vi "Add Item Buffered.vi"(8 "错误输入":errorcluster, 9 "Length":i32=20, 10 "Item":string[](array[string]), 11 "Mlistbox Ref":refnum<vi>) -> (0 "错误输出":errorcluster, 3 "Mlistbox Ref Dup":refnum<vi>)   [LabVIEW 2012, in "Mlistbox Tools.lvlib"]
uses:
  Mlistbox Tools.lvlib
  ListBox/Custom Type/Read and Write Mode.ctl
  Property/Set and Get ItemNames.vi
  ListBox/Listbox Tool.lvlib
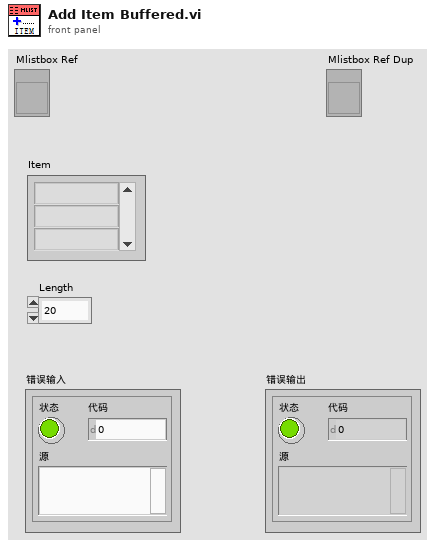
[diagram p1: front panel]
types:
  T1 = typedef "Listbox Tool.lvlib/Read and Write Mode.ctl" = enum16{"Read", "Write"}
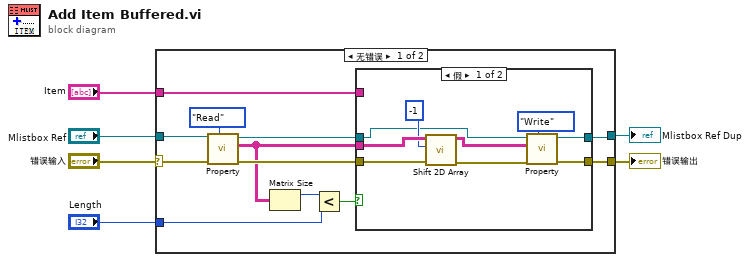
[diagram p0: block diagram]
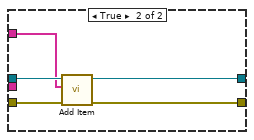
[diagram p2: hidden frame]
diagram:
  n1 = case shown="无错误" "错误输入" {
    selector: "错误输入" -> [w16 w34]
    tunnel: [w8 w34] -> w5
    tunnel: "Mlistbox Ref" -> [w18 w33]
    tunnel: "Item" -> [w10 _]
    tunnel: [w9 w33] -> w2
    tunnel: "Length" -> [w14 _]
    frame No Error {
      n2 = call-poly "Property.vi"("Mode"=Read_and_Write_Mode."Read", "错误输入"=w16, "Mlistbox Ref"=w18) -> ("错误输出"=w12:errorcluster, "ItemNames Out"=w7:string[][], "Mlistbox Ref Dup"=w11:refnum<vi>)  [unwired: 6 in]
      n3 = Matrix Size(0:w7) -> (1:w15:i32)  [unwired: 1 out]
      n4 = Less?(x=w15, y=w14) -> (x < y?=w13:bool)
      n5 = case shown="假" w13 {
        tunnel: w12 -> [w27 w32]
        tunnel: w11 -> [w24 w31]
        tunnel: w10 -> [_ w30]
        tunnel: [w20 w29] -> w9
        tunnel: [w19 w28] -> w8
        tunnel: w7 -> [w26 _]
        frame False {
          n6 = call-poly "Shift 2D Array.vi"("error in (no error)"=w27, "n"=-1, "Input Array"=w26) -> ("error out"=w22:errorcluster, "Output Array"=w23:string[][])  [unwired: 7 in]
          n7 = call-poly "Property.vi"("Mode"=Read_and_Write_Mode."Write", "错误输入"=w22, "ItemNames In"=w23, "Mlistbox Ref"=w24) -> ("错误输出"=w19:errorcluster, "Mlistbox Ref Dup"=w20:refnum<vi>)  [unwired: 5 in, 1 out]
        }
        frame True {
          n8 = call "Add Item.vi"("错误输入"=w32, "Item"=w30, "Mlistbox Ref"=w31) -> ("错误输出"=w28:errorcluster, "Mlistbox Ref Dup"=w29:refnum<vi>)  [unwired: 7 in]
        }
      }
    }
    frame Error {
    }
  }
  "Mlistbox Ref Dup" <- w2
  "错误输出" <- w5
